vi "Converge.vi"(7 "Fractal type":enum16{"Mandelbrot", "Julia"}(ring), 9 "Z0":cdb, 10 "Iterations":i32, 11 "C":cdb) -> (2 "IN":bool, 3 "Numeric":i32)   [LabVIEW 2015]
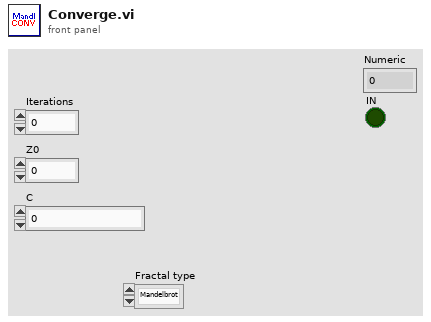
[diagram p1: front panel]
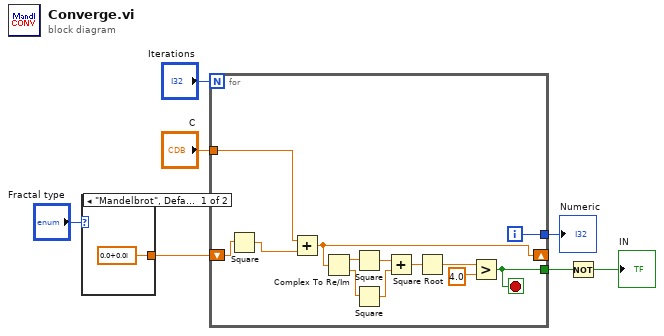
[diagram p0: block diagram]
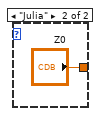
[diagram p2: hidden frame]
diagram:
  n1 = case shown="\"Mandelbrot\", Default" "Fractal type" {
    tunnel: [cdb 0.0+0.0i ("r * e^(i*theta)") "Z0"] -> w1
    frame "Mandelbrot", Default {
    }
    frame "Julia" {
    }
  }
  n2 = for {
    N: "Iterations" -> [_]
    shift-right: [w14] -> _
    shift-left: w1 -> [w11]
    tunnel: "C" -> [w22]
    tunnel: [w13] -> w5
    tunnel: [w12] -> w4
    i -> [w13]
    stop <- w12 stop-if-true
    n3 = Square(x=w11) -> (x^2=w10:cdb)
    n4 = Add(x=w22, y=w10) -> (x+y=w14:cdb)
    n5 = Complex To Re/Im(x + iy=w14) -> (x=w20:dbl, y=w21:dbl)
    n6 = Square(x=w20) -> (x^2=w19:dbl)
    n7 = Square(x=w21) -> (x^2=w18:dbl)
    n8 = Add(x=w19, y=w18) -> (x+y=w17:dbl)
    n9 = Square Root(x=w17) -> (sqrt(x)=w16:dbl)
    n10 = Greater?(x=w16, y=4.0) -> (0:w12:bool)
  }
  "Numeric" <- w5
  n11 = Not(x=w4) -> (.not. x?=→"IN":bool)
